vi "Logger_Do.vi"(8 "error in (no error)":errorcluster caption="错误输入（无错误）", 10 "Message":T1, 11 "Logger 输入":refnum<class "Logger.lvclass">) -> (0 "error out":errorcluster caption="错误输出", 3 "Logger 输出":refnum<class "Logger.lvclass">)   [LabVIEW 2019, in "Logger.lvclass"]
uses:
  <userlib>/Logger/Logger.lvclass
  <userlib>/Logger/Ctls/LoggerMessage.ctl
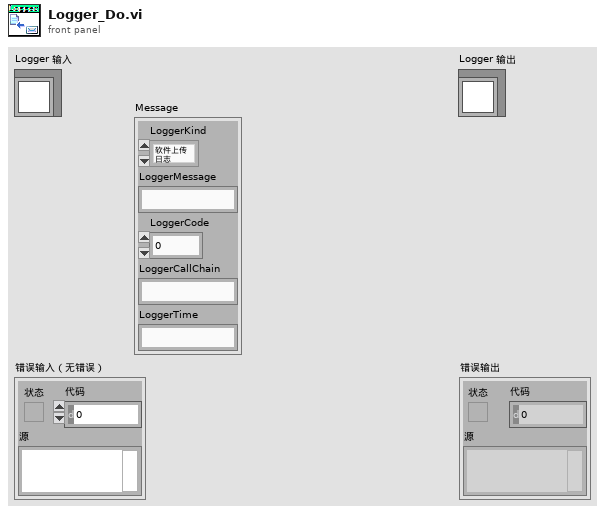
[diagram p1: front panel]
types:
  T1 = typedef "Logger.lvclass/LoggerMessage.ctl" = cluster{"LoggerKind":enum16{"软件上传日志", "软件其他日志", "软件错误日志", "软件监控日志"}, "LoggerMessage":string, "LoggerCode":i32, "LoggerCallChain":string, "LoggerTime":string}
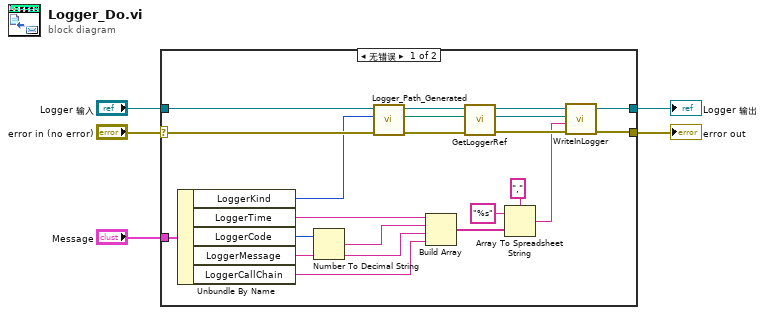
[diagram p0: block diagram]
diagram:
  n1 = case shown="无错误" "error in (no error)" {
    selector: "error in (no error)" -> [w14 w26]
    tunnel: [w6 w26] -> w4
    tunnel: [w10 w25] -> w2
    tunnel: "Logger 输入" -> [w24 w25]
    tunnel: "Message" -> [w23 _]
    frame No Error {
      n2 = Unbundle By Name(w23) -> ("LoggerKind"=w13:enum16{"软件上传日志", "软件其他日志", "软件错误日志", "软件监控日志"}, "LoggerTime"=w21:string, "LoggerCode"=w22:i32, "LoggerMessage"=w19:string, "LoggerCallChain"=w15:string)
      n3 = Number To Decimal String(number=w22) -> (decimal integer string=w20:string)  [unwired: 1 in]
      n4 = call <userlib>:"Logger_Path_Generated.vi"("error in (no error)"=w14, "LoggerKind"=w13, "Logger 输入"=w24) -> ("error out"=w12:errorcluster, "appended path"=w11:path, "Logger 输出"=w10:refnum<class "Logger.lvclass">)  [unwired: 6 in]
      n5 = Build Array(w21, w20, w19, w15) -> (w18:string[])
      n6 = call <userlib>:"GetLoggerRef.vi"("error in (no error)"=w12, "LoggerSavePath"=w11) -> ("error out"=w9:errorcluster, "refnum"=w8:refnum<file>)  [unwired: 8 in]
      n7 = Array To Spreadsheet String(delimiter (Tab)="," ("分隔符(Tab)"), array=w18, 3:"%s" ("格式字符串")) -> (spreadsheet string=w7:string)
      n8 = call <userlib>:"WriteInLogger.vi"("错误输入"=w9, "LoggerData"=w7, "refnum"=w8) -> ("错误输出"=w6:errorcluster)  [unwired: 8 in]
    }
    frame Error {
    }
  }
  "error out" <- w4
  "Logger 输出" <- w2
